vi "Set Feedback Sig Parametes.vi"(8 "error in (no error)":errorcluster, 9 "Encoder Const (1)":i32=1, 10 "Channel":i32(ring)=1 items=["Channel1"=1, "Channel2"=2, "Channel3"=3, "Channel4"=4], 11 "Device in":refnum<k24>) -> (0 "error out":errorcluster, 3 "Device out":refnum<k24>)   [LabVIEW 2017, in "XYStage.KIM101.lvclass"]
uses:
  XYStage.KIM101.lvclass
  C:/Program Files (x86)/Thorlabs/Kinesis/Thorlabs.MotionControl.KCube.InertialMotorCLI.dll
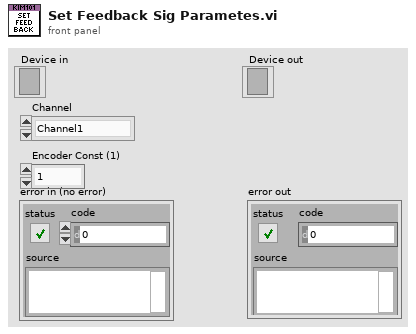
[diagram p1: front panel]
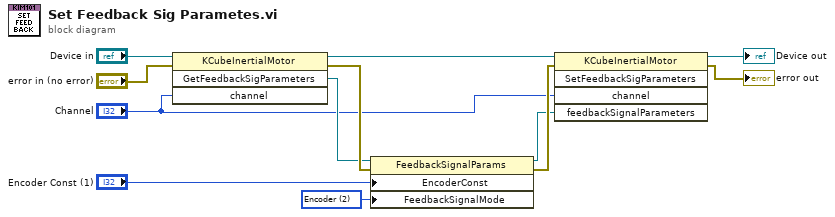
[diagram p0: block diagram]
diagram:
  w11 = 2 items=["Disabled", "LimitSwitch", "Encoder"] ("FeedbackSignalMode")
  n1 = invoke class="KCubeInertialMotor" method="GetFeedbackSigParameters"(reference="Device in", error in="error in (no error)", "channel"="Channel") -> (reference out=w9:refnum<k24>, error out=w12:errorcluster, "GetFeedbackSigParameters"=w10:refnum<k24>)  [unwired: 1 in, 1 out]
  n2 = property class="FeedbackSignalParams"(reference=w10, error in=w12, "EncoderConst"="Encoder Const (1)", "FeedbackSignalMode"=w11) -> (reference out=w7:refnum<k24>, error out=w8:errorcluster)
  n3 = invoke class="KCubeInertialMotor" method="SetFeedbackSigParameters"(reference=w9, error in=w8, "channel"="Channel", "feedbackSignalParameters"=w7) -> (reference out=→"Device out":refnum<k24>, error out=→"error out":errorcluster)  [unwired: 1 in, 3 out]
